vi "SLSC Create Commands.vi"(11 "RevA?":bool) -> (3 "Outgoing configuration":T3(array[cluster])=[{"Channel Name"="LED1_Green", "SLSC Name"="Bool.LED1.NI.GreenBool", "Channel"={"Type"=enum."Input", "Units"="", "Default Value"=1.0, "Faultable"=FALSE, "Scalable"=FALSE}}, {"Channel Name"="Scratchpad8", "SLSC Name"="U32.Scratchpad8.NI.Scratchpad.AsUInt32.U8", "Channel"={"Type"=enum."Input", "Units"="", "Default Value"=12.0, "Faultable"=FALSE, "Scalable"=FALSE}}])   [LabVIEW 2015, in "SLSC-12201 DIO System Explorer.lvlib"]
uses:
  SLSC-12201 DIO System Explorer.lvlib
  <vilib>/NI Veristand/Custom Device API/Custom Device Channel.ctl
  <vilib>/NI Veristand/Custom Device API/Custom Device Channel Type.ctl
  <vilib>/NI Veristand/Custom Device API/Custom Device API.lvlib
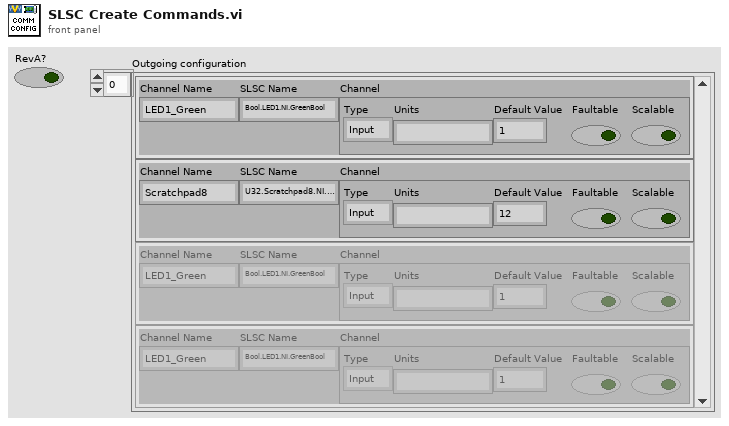
[diagram p1: front panel]
types:
  T1 = typedef "Custom Device API.lvlib/Custom Device Channel.ctl" = cluster{"Type":T2, "Units":string, "Default Value":dbl, "Faultable":bool, "Scalable":bool}
  T2 = typedef "Custom Device API.lvlib/Custom Device Channel Type.ctl" = enum16{"Input", "Output"}
  T3 = cluster{"Channel Name":string, "SLSC Name":string, "Channel":T1}[]
  T4 = cluster{"Channel Name":string, "SLSC Name":string, "Configuration":T1}[]
  T5 = cluster{"Channel Name":string, "SLSC Name":string, "Configuration":T1}
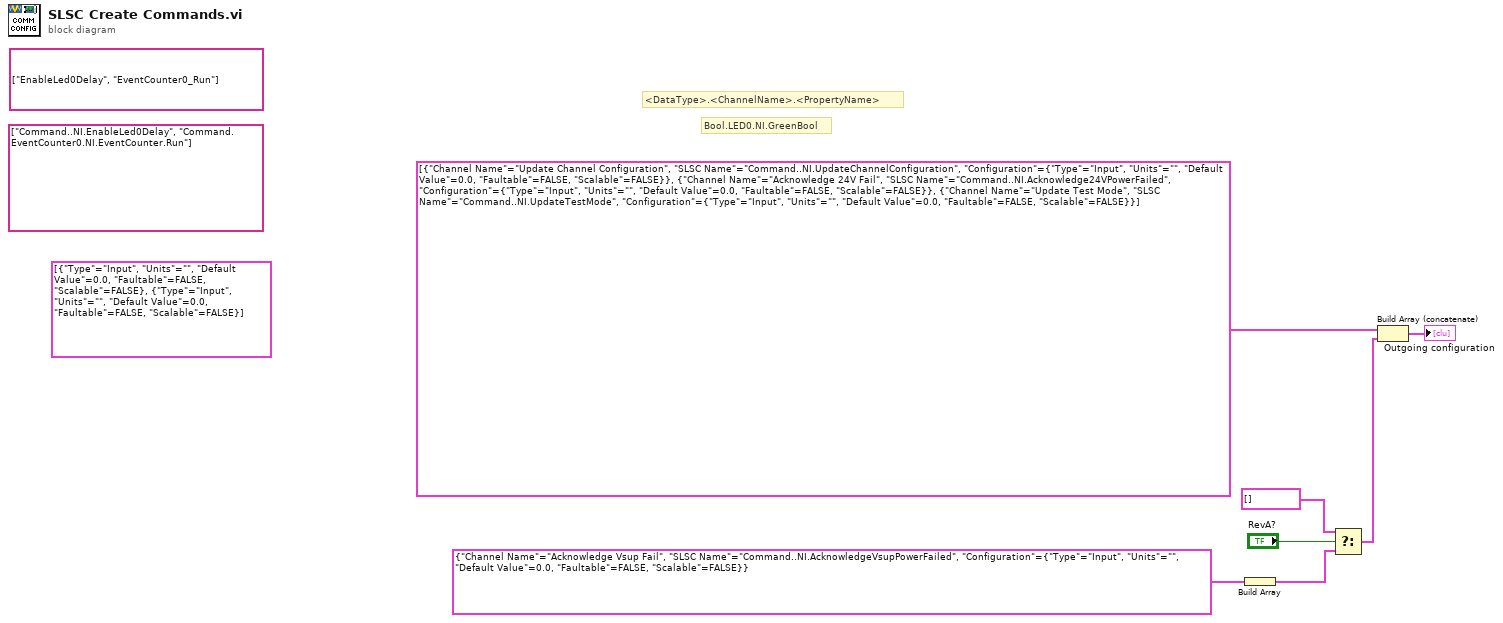
[diagram p0: block diagram]
diagram:
  (unwired) T1[] [{"Type"=enum."Input", "Units"="", "Default Value"=0.0, "Faultable"=FALSE, "Scalable"=FALSE}, {"Type"=enum."Input", "Units"="", "Default Value"=0.0, "Faultable"=FALSE, "Scalable"=FALSE}]
  (unwired) string[] ["EnableLed0Delay", "EventCounter0_Run"]
  (unwired) string[] ["Command..NI.EnableLed0Delay", "Command.EventCounter0.NI.EventCounter.Run"]
  # "Bool.LED0.NI.GreenBool"
  # "<DataType>.<ChannelName>.<PropertyName>"
  n1 = Build Array(T5 {"Channel Name"="Acknowledge Vsup Fail", "SLSC Name"="Command..NI.AcknowledgeVsupPowerFailed", "Configuration"={"Type"=enum."Input", "Units"="", "Default Value"=0.0, "Faultable"=FALSE, "Scalable"=FALSE}}) -> (w3:T4)
  n2 = Select(t=T4 [], s="RevA?", f=w3) -> (s? t:f=w1:T4)
  n3 = Build Array (concatenate)(T4 [{"Channel Name"="Update Channel Configuration", "SLSC Name"="Command..NI.UpdateChannelConfiguration", "Configuration"={"Type"=enum."Input", "Units"="", "Default Value"=0.0, "Faultable"=FALSE, "Scalable"=FALSE}}, {"Channel Name"="Acknowledge 24V Fail", "SLSC Name"="Command..NI.Acknowledge24VPowerFailed", "Configuration"={"Type"=enum."Input", "Units"="", "Default Value"=0.0, "Faultable"=FALSE, "Scalable"=FALSE}}, {"Channel Name"="Update Test Mode", "SLSC Name"="Command..NI.UpdateTestMode", "Configuration"={"Type"=enum."Input", "Units"="", "Default Value"=0.0, "Faultable"=FALSE, "Scalable"=FALSE}}], w1) -> (→"Outgoing configuration":T4)
